vi "segment time.vi"(4 "Intial time t(0)":u32, 5 "segment time t(i-1)":dbl[](array[numeric]) format="%#_9g") -> (0 "% time oqupied":dbl[](array[numeric]) format="%#.2g", 1 "total time t(i)":dbl, 2 "segment time t(i)-t(i-1)":dbl[](array[numeric]) format="%.3g")   [LabVIEW 2016]
panel:
  out "x/y":dbl[](array[numeric])
  out "Last time(ms)":u32
  # "0"
  # "0"
  # "0"
  # "1"
  # "1"
  # "1"
  # "2"
  # "2"
  # "2"
  # "3"
  # "3"
  # "3"
  # "4"
  # "4"
  # "4"
  # "5"
  # "5"
  # "5"
  # "end"
  # "end"
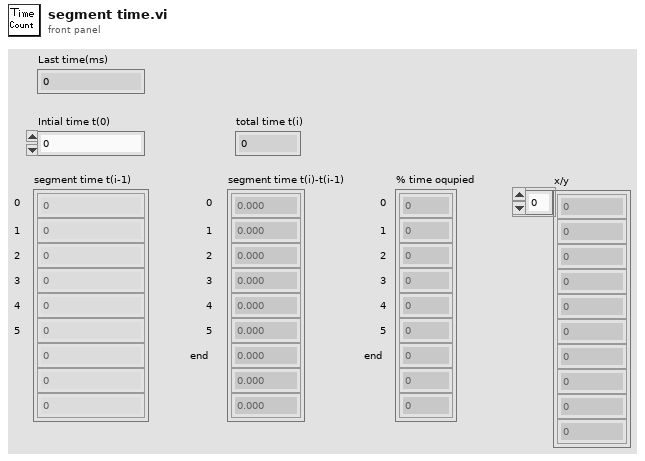
[diagram p1: front panel]
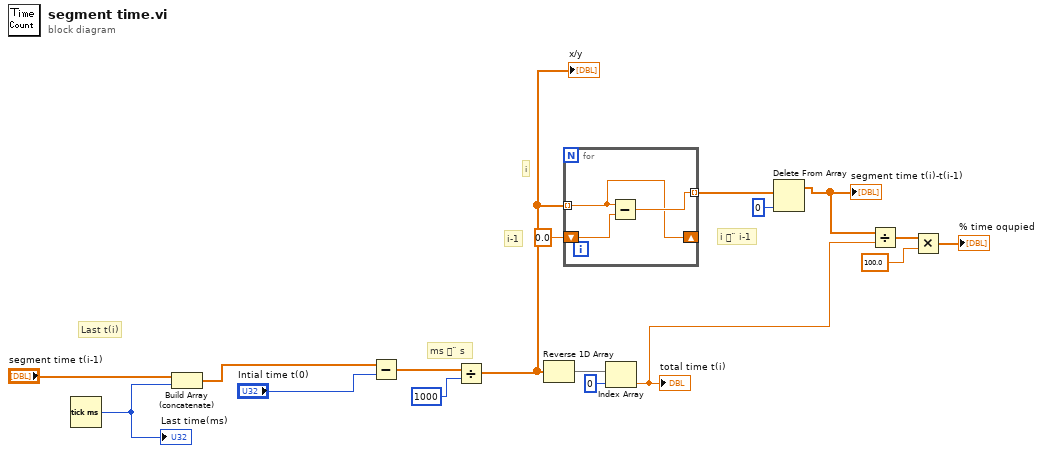
[diagram p0: block diagram]
diagram:
  # "i ¨ i-1"
  # "i"
  # "i-1"
  # "Last t(i)"
  # "ms ¨ s"
  n1 = Tick Count (ms)() -> (millisecond timer value=w1:u32)
  "Last time(ms)" <- w1
  n2 = Build Array (concatenate)("segment time t(i-1)", w1) -> (w13:dbl[])
  n3 = Subtract(x=w13, y="Intial time t(0)") -> (x-y=w15:dbl[])
  n4 = Divide(x=w15, y=u32 1000) -> (x/y=w10:dbl[])
  "x/y" <- w10
  n5 = Reverse 1D Array(array=w10) -> (reversed array=w12:dbl[])
  n6 = for {
    tunnel: w10 -> [w19] mode=indexing
    shift-right: [w19] -> _
    shift-left: 0.0 ("y") -> [w18]
    tunnel: [w20] -> w4 mode=indexing
    n7 = Subtract(x=w19, y=w18) -> (x-y=w20:dbl)
  }
  n8 = Index Array(array=w12, index=0 ("指標")) -> (element=w8:dbl)
  "total time t(i)" <- w8
  n9 = Delete From Array(array=w4, index=0 ("指標")) -> (array with subset deleted=w2:dbl[])  [unwired: 1 in, 1 out]
  "segment time t(i)-t(i-1)" <- w2
  n10 = Divide(x=w2, y=w8) -> (x/y=w7:dbl[])
  n11 = Multiply(x=w7, y=100.0) -> (x*y=→"% time oqupied":dbl[])
